vi "Config System Actors.vi"(8 "error in (no error)":errorcluster, 10 "Root Actor In":refnum<class "Root Actor.lvclass">, 11 "System Modules Factory in":refnum<class "System Modules Factory.lvclass">) -> (0 "error out":errorcluster, 2 "Root Actor Out":refnum<class "Root Actor.lvclass">, 3 "System Modules Factory out":refnum<class "System Modules Factory.lvclass">)   [LabVIEW 2024, in "System Modules Factory.lvclass"]
uses:
  System Modules Factory.lvclass
  Actor/Root Actor/Root Actor.lvclass
  System Modules Factory.lvclass/System Modules Factory.ctl
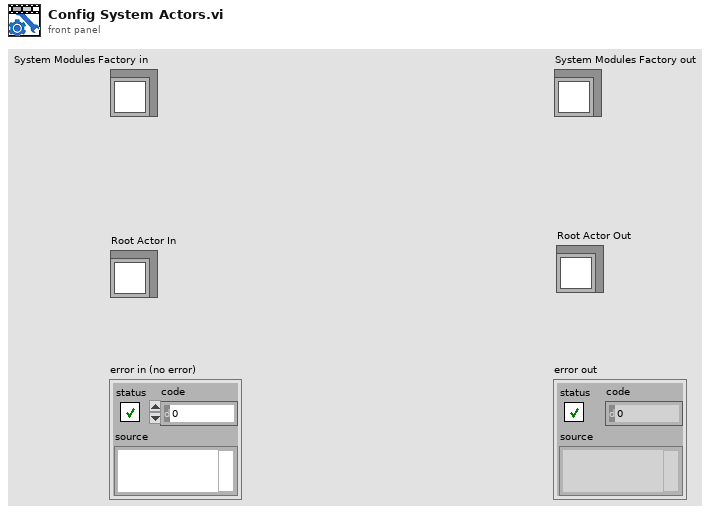
[diagram p1: front panel]
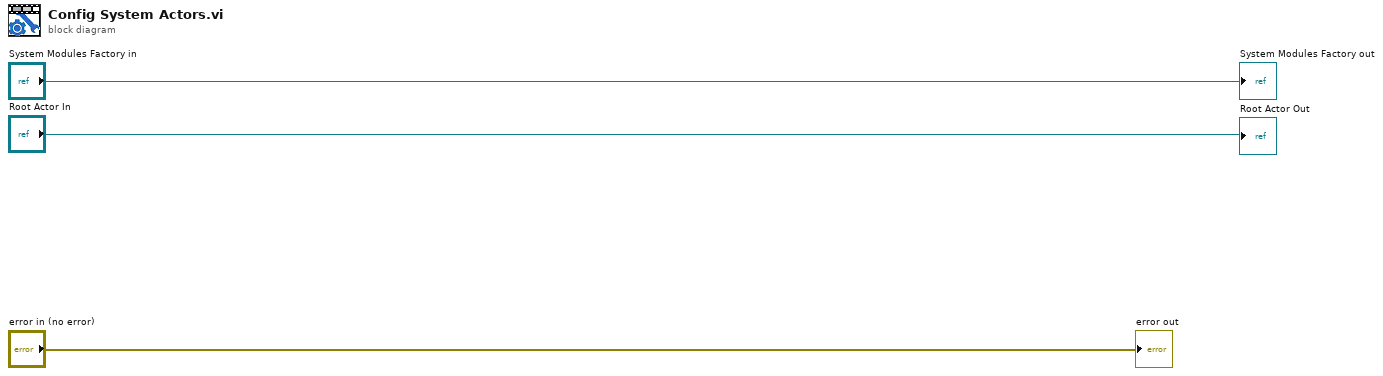
[diagram p0: block diagram]
diagram:
  "error out" <- "error in (no error)"
  "System Modules Factory out" <- "System Modules Factory in"
  "Root Actor Out" <- "Root Actor In"
